vi "CRYMake New Group Dialog.vi"(11 "Type":enum16{"Curves", "Values", "Results", "WFM"}(ring)) -> (0 "Return Flag":bool, 1 "Org Group Name":string caption="aa", 2 "InGroup?":bool caption="Group?", 3 "New Group Name":string caption="aa")   [LabVIEW 2013]
panel:
  in  "Group Name":string caption="aa"
  in  "Cancel":bool
  in  "OK":bool
  in  "Group":bool caption="Group Selected Items"
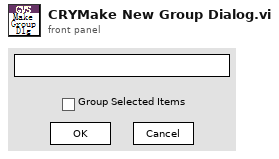
[diagram p1: front panel]
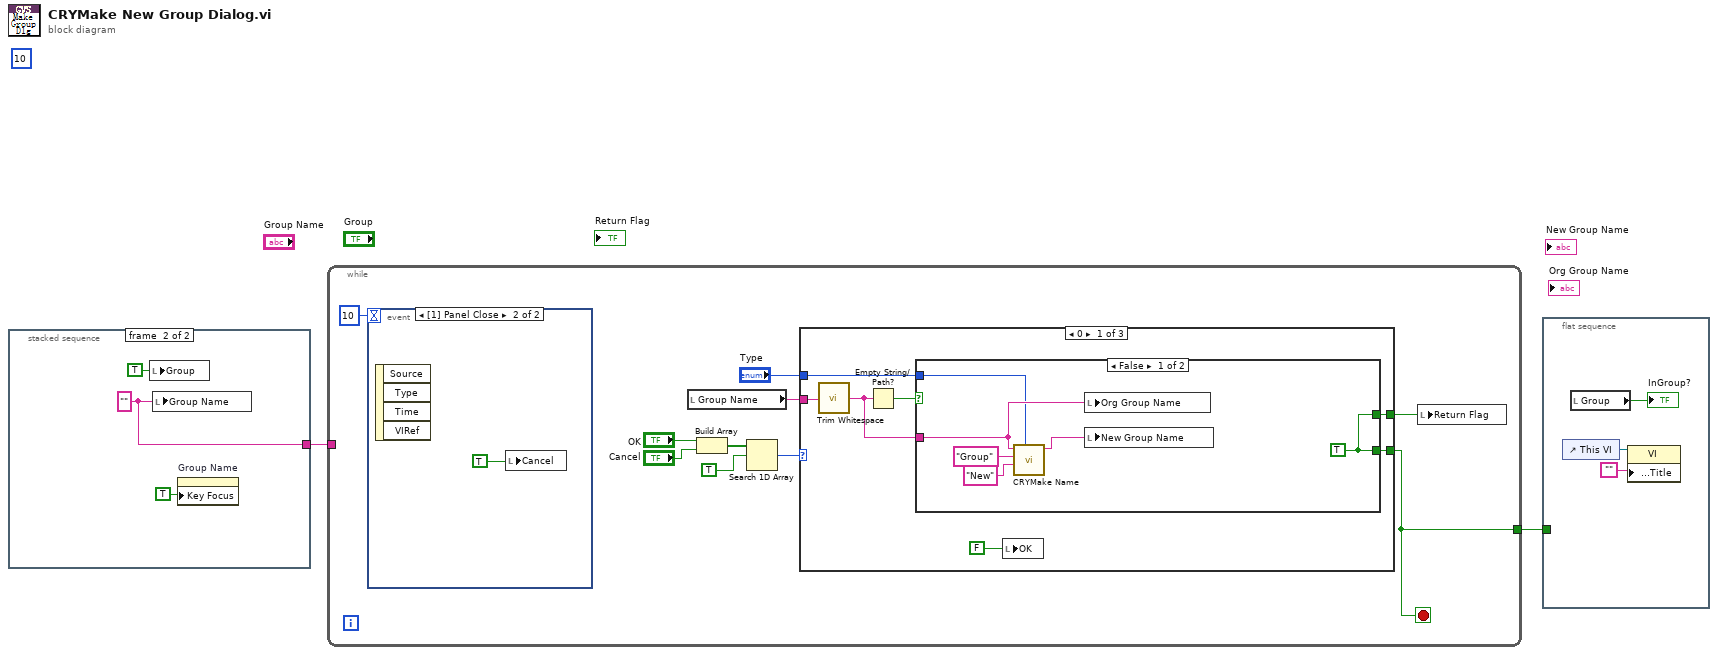
[diagram p0: block diagram]
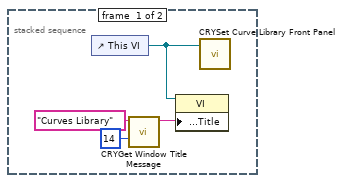
[diagram p2: hidden frame]
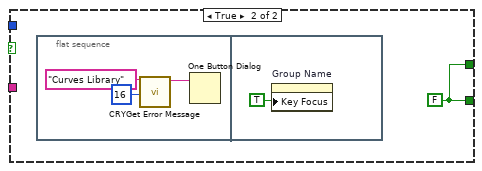
[diagram p3: hidden frame]
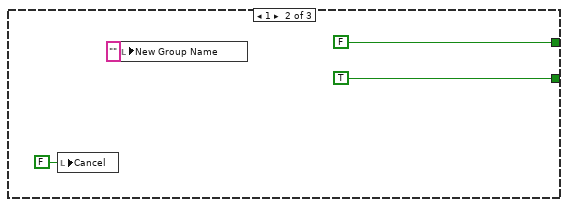
[diagram p4: hidden frame]
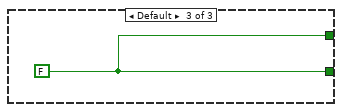
[diagram p5: hidden frame]
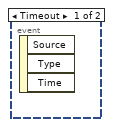
[diagram p6: hidden frame]
diagram:
  (unwired) 10
  n1 = stacked-sequence {
    tunnel: [_ w8] -> w2
    frame #0 {
      n2 = control-ref of="This VI"() -> (w6:refnum<vi>)
      n3 = call "CRYGet Window Title Message.vi"("No"=14 ("Error No"), "Kind"="Curves Library") -> ("Multibyte String"=w3:string)  [unwired: 4 in, 5 out]
      n4 = property class="VI"(reference=w6, "Front Panel.Title"=w3) -> ()  [unwired: 1 in, 2 out]
      n5 = call "CRYSet Curve Library Front Panel.vi"("Vi Ref In"=w6) -> ()  [unwired: 10 in, 1 out]
    }
    frame #1 {
      w8 = "" ("Group Name")
      n6 = local write "Group"(TRUE ("Group")) -> ()
      n7 = local write "Group Name"(w8) -> ()
      n8 = property on="Group Name" class="Str"("Key Focus"=TRUE) -> ()  [unwired: 2 in, 2 out]
    }
  }
  n9 = while {
    tunnel: [w13] -> w1
    tunnel: w2 -> [_]
    stop <- w13 stop-if-true
    n10 = event shown="[1] Panel Close" {
      selector: _ -> [_ _]
      dyn-events: _ -> [_ _]
      timeout: 10 -> [_ _]
      event Timeout {
        n11 = event-data() -> ()  [unwired: 1 in, 3 out]
      }
      event Panel Close {
        n12 = event-data() -> ()  [unwired: 1 in, 4 out]
        n13 = local write "Cancel"(TRUE) -> ()
      }
    }
    n14 = local read "Group Name"() -> (w12:string)
    n15 = Build Array("OK", "Cancel") -> (w17:bool[])
    n16 = Search 1D Array(1D array=w17, element=TRUE) -> (index of element=w14:i32)  [unwired: 1 out]
    n17 = case shown="0" w14 {
      tunnel: [w22 TRUE ("Cancel") w42] -> w13
      tunnel: w12 -> [w25 _ _]
      tunnel: [w21 FALSE ("Cancel") w42] -> w11
      tunnel: "Type" -> [w20 _ _]
      frame 0 {
        n18 = call <vilib>:"Trim Whitespace.vi"("string"=w25) -> ("trimmed string"=w23:string)  [unwired: 1 in]
        n19 = Empty String/Path?(string/path=w23) -> (empty?=w24:bool)
        n20 = case shown="False" w24 {
          tunnel: w23 -> [w28 _]
          tunnel: [w32 w33] -> w22
          tunnel: [w32 w33] -> w21
          tunnel: w20 -> [w27 _]
          frame False {
            w32 = TRUE ("Cancel")
            n21 = call "CRYMake Name.vi"("Type"=w27, "sOption"="New", "sAction"="Group", "Name In"=w28) -> ("Name Out"=w30:string)  [unwired: 6 in, 1 out]
            n22 = local write "Org Group Name"(w28) -> ()
            n23 = local write "New Group Name"(w30) -> ()
          }
          frame True {
            w33 = FALSE ("Cancel")
            n24 = flat-sequence {
              frame #0 {
                n25 = call "CRYGet Error Message.vi"("Error No"=16 ("No"), "Kind"="Curves Library") -> ("Message"=w34:string)  [unwired: 4 in, 5 out]
                n26 = One Button Dialog(message=w34) -> ()  [unwired: 2 out]
              }
              frame #1 {
                n27 = property on="Group Name" class="Str"("Key Focus"=TRUE) -> ()  [unwired: 2 in, 2 out]
              }
            }
          }
        }
        n28 = local write "OK"(FALSE ("Cancel")) -> ()
      }
      frame 1 {
        n29 = local write "Cancel"(FALSE ("Cancel")) -> ()
        n30 = local write "New Group Name"("" ("Group Name")) -> ()
      }
      frame Default {
        w42 = FALSE ("Cancel")
      }
    }
    n31 = local write "Return Flag"(w11) -> ()
  }
  n32 = flat-sequence {
    tunnel: w1 -> [_]
    frame #0 {
      n33 = control-ref of="This VI"() -> (w46:refnum<vi>)
      n34 = local read "Group"() -> (→"InGroup?":bool)
      n35 = property class="VI"(reference=w46, "Front Panel.Title"="") -> ()  [unwired: 1 in, 2 out]
    }
  }
